vi "GetDefaultParams.vi"(8 "error in (no error)":errorcluster, 10 "Path":path, 11 "FgenPluginsBase in":refnum<class "FgenPluginsBase.lvclass">) -> (0 "error out":errorcluster, 3 "FgenPluginsBase out":refnum<class "FgenPluginsBase.lvclass">)   [LabVIEW 2018, in "FgenPlugins.lvlib" / "FgenPluginsBase.lvclass"]
uses:
  FgenPluginsBase.lvclass
  C:/Program Files (x86)/National Instruments/LabVIEW 2018/user.lib/NIST/BaseClasses/BasePlugin_class/BasePlugin.lvclass
  TypeDefs/Channels.ctl
  TypeDefs/Channel.ctl
  TypeDefs/clTriggers.ctl
  TypeDefs/Trigger.ctl
  TypeDefs/TriggerType.ctl
  MemberClasses/FunctionBaseClass/FunctionBase.lvclass
  <userlib>/NIST/BaseClasses/BasePlugin_class/BasePlugin.lvclass/BasePlugin.ctl
  FgenPluginsBase.lvclass/FgenPluginsBase.ctl
  <userlib>/NIST/BaseClasses/BasePlugin_class/Accessors/Write PluginIniFilePath.vi
  Accessors/Write Channels.vi
  Accessors/Write FunctionINIFilePath.vi
  Accessors/Write FunctionClass.vi
  Accessors/Write Triggers.vi
  <vilib>/Utility/error.llb/Error Cluster From Error Code.vi
  <vilib>/ErrorRing/Error Ring.xnode
  <vilib>/Utility/config.llb/NI_LVConfig.lvlib
  FgenPlugins.lvlib
  <userlib>/NIST/BaseClasses/Object_class/BaseObject.lvclass
panel:
  out "Path":path
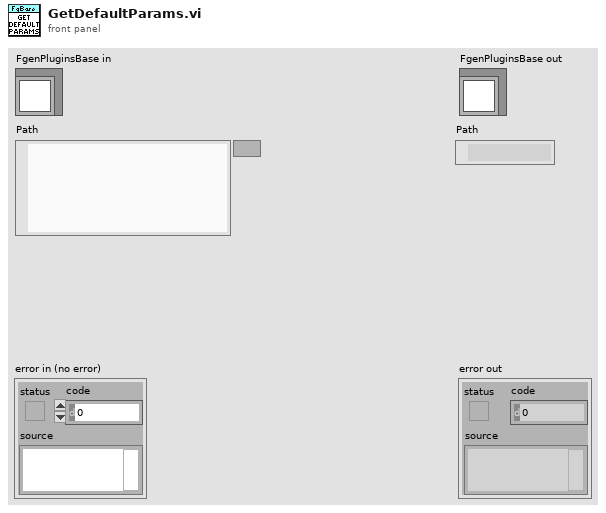
[diagram p1: front panel]
types:
  T1 = typedef "FgenPlugins.lvlib/clTriggers.ctl" = cluster{"Count":i32, "Triggers":T2[]}
  T2 = typedef "FgenPlugins.lvlib/Trigger.ctl" = cluster{"Source":string, "Slope":enum16{"Positive", "Negative", "Either"}, "Threshold":dbl, "Delay":dbl, "TriggerType":T3}
  T3 = typedef "FgenPlugins.lvlib/TriggerType.ctl" = enum16{"None", "Start", "Stop", "Hold", "Resume", "Advance"}
  T4 = typedef "FgenPlugins.lvlib/Channels.ctl" = cluster{"Count":u16, "Channel":T5[]}
  T5 = typedef "FgenPlugins.lvlib/Channel.ctl" = cluster{"Name":string, "Enabled":bool, "Operation":enum16{"Continuous", "Burst"}, "Impedance (50)":dbl, "Handle":string, "Connected":bool, "Mode (Function)":enum16{"Function", "Arbitrary", "Sequence"}}
  T6 = typedef "NI_LVConfig.lvlib/Config Data RefNum.ctl" = refnum<k1>
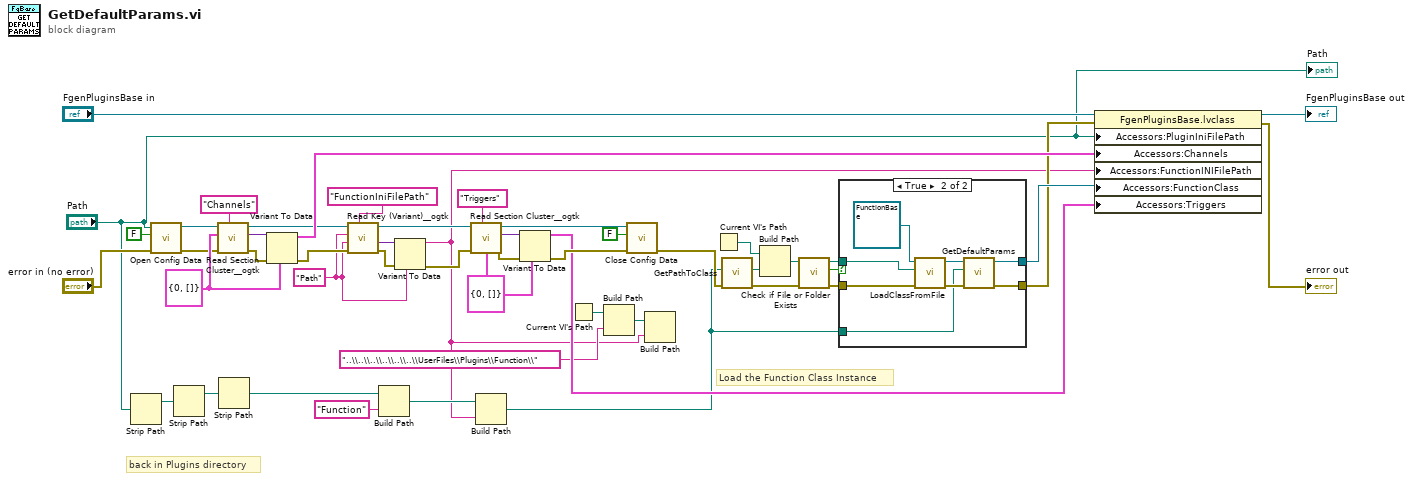
[diagram p0: block diagram]
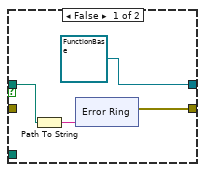
[diagram p2: hidden frame]
diagram:
  w12 = T1 {"Count"=0, "Triggers"=[]} ("Triggers")
  w21 = "Path" ("key (optional)")
  w43 = T4 {"Count"=0, "Channel"=[]} ("Channels")
  # "back in Plugins directory"
  # "Load the Function Class Instance"
  n1 = Strip Path(path="Path") -> (stripped path=w7:path)  [unwired: 1 out]
  n2 = call <vilib>:"Open Config Data.vi"("error in (no error)"="error in (no error)", "create file if necessary (T)"=FALSE, "configuration file path"="Path") -> ("error out"=w39:errorcluster, "refnum"=w44:T6)  [unwired: 6 in, 1 out]
  n3 = Strip Path(path=w7) -> (stripped path=w6:path)  [unwired: 1 out]
  n4 = call <userlib>:"Read Section Cluster__ogtk.vi"("section (optional)"="Channels", "error in (no error)"=w39, "Section Formatted Cluster Type"=w43, "refnum"=w44) -> ("error out"=w38:errorcluster, "Section Formatted Cluster"=w48:variant, "dup refnum"=w36:T6)  [unwired: 3 in, 2 out]
  n5 = Strip Path(path=w6) -> (stripped path=w1:path)  [unwired: 1 out]
  n6 = Variant To Data(error in=w38, type=w43, Variant=w48) -> (data=w41:T4, error out=w35:errorcluster)
  n7 = call <userlib>:"Read Key (Variant)__ogtk.vi"("section"="FunctionIniFilePath", "error in (no error)"=w35, "type"=w21, "key (optional)"=w21, "refnum"=w36) -> ("error out"=w32:errorcluster, "key-value"=w33:variant, "refnum out"=w18:T6)  [unwired: 3 in, 1 out]
  n8 = Build Path(base path=w1, name or relative path="Function") -> (appended path=w4:path)
  n9 = Variant To Data(error in=w32, type=w21, Variant=w33) -> (data=w3:string, error out=w19:errorcluster)
  n10 = call <userlib>:"Read Section Cluster__ogtk.vi"("section (optional)"="Triggers", "error in (no error)"=w19, "Section Formatted Cluster Type"=w12, "refnum"=w18) -> ("error out"=w15:errorcluster, "Section Formatted Cluster"=w14:variant, "dup refnum"=w17:T6)  [unwired: 3 in, 2 out]
  n11 = Build Path(base path=w4, name or relative path=w3) -> (appended path=w2:path)
  n12 = Variant To Data(error in=w15, type=w12, Variant=w14) -> (data=w11:T1, error out=w13:errorcluster)
  n13 = Current VI's Path() -> (path=w20:path)
  n14 = Build Path(base path=w20, name or relative path="..\\..\\..\\..\\..\\..\\UserFiles\\Plugins\\Function\\") -> (appended path=w9:path)
  n15 = call <vilib>:"Close Config Data.vi"("error in (no error)"=w13, "write file if changed (T)"=FALSE, "refnum"=w17) -> ("error out"=w24:errorcluster)  [unwired: 7 in, 1 out]
  n16 = Build Path(base path=w9, name or relative path=w3) -> ()  [unwired: 1 out]
  n17 = Current VI's Path() -> (path=w26:path)
  n18 = call <userlib>:"GetPathToClass.vi"("error in (no error)"=w24, "configuration file path"=w2) -> ("error IO"=w29:errorcluster, "PathToClass"=w27:path)  [unwired: 8 in]
  n19 = Build Path(base path=w26, name or relative path=w27) -> (appended path=w25:path)
  n20 = call <vilib>:"Check if File or Folder Exists.vi"("error in (no error)"=w29, "path"=w25) -> ("error out"=w30:errorcluster, "file or folder exists?"=w28:bool, "dup path"=w31:path)  [unwired: 7 in]
  n21 = case shown="True" w28 {
    tunnel: [w52 w63] -> w22
    tunnel: w30 -> [_ w68]
    tunnel: w31 -> [w51 w67]
    tunnel: w2 -> [_ w61]
    tunnel: [refnum<class "FunctionBase.lvclass"> refnum ("Functions.lvlib:FunctionBase.lvclass") w62] -> w23
    frame False {
      n22 = Path To String(path=w51) -> (string=w53:string)
      n23 = xnode "Error Ring"("parameter 0"=w53) -> ("error out"=w52:errorcluster)
    }
    frame True {
      n24 = call-dynamic "LoadClassFromFile.vi"("error in (no error)"=w68, "class path"=w67, "reference in"=refnum<class "FunctionBase.lvclass"> refnum ("Functions.lvlib:FunctionBase.lvclass")) -> ("error out"=w65:errorcluster, "reference out"=w64:refnum<class "FunctionBase.lvclass">)  [unwired: 7 in]
      n25 = call-dynamic "GetDefaultParams.vi"("error in (no error)"=w65, "Path"=w61, "FunctionBase in"=w64) -> ("error out"=w63:errorcluster, "FunctionBase out"=w62:refnum<class "FunctionBase.lvclass">)  [unwired: 7 in]
    }
  }
  n26 = property class="FgenPluginsBase.lvclass"(reference="FgenPluginsBase in", error in=w22, "Accessors:PluginIniFilePath"="Path", "Accessors:Channels"=w41, "Accessors:FunctionINIFilePath"=w3, "Accessors:FunctionClass"=w23, "Accessors:Triggers"=w11) -> (reference out=→"FgenPluginsBase out":refnum<class "FgenPluginsBase.lvclass">, error out=→"error out":errorcluster)
  "Path" <- "Path"
